vi "Wait.vi"(11 "Time (ms)":u32) -> (3 "Node Out":refnum<class "bt_Node.lvclass">)   [LabVIEW 2021, in "BT.lvlib"]
uses:
  BT.lvlib
  Support/Nodes/abs_Node/bt_Node.lvclass
  Support/Nodes/Leaves/Wait/bt_Wait.lvclass
  C:/Users/Tim/Documents/GitHub/LV_Behaviour_Tree/Source/Support/Nodes/abs_Node/BT_Node.lvclass
  Support/Nodes/Leaves/Wait/bt_Wait.lvclass/bt_Wait.ctl
  Support/Nodes/Leaves/Wait/Properties/Write Time (ms).vi
  C:/Users/Tim/Documents/GitHub/LV_Behaviour_Tree/Source/Support/Nodes/Leaves/Leaf/bt_Leaf.lvclass
  C:/Users/Tim/Documents/GitHub/LV_Behaviour_Tree/Source/Support/Nodes/abs_Node/bt_Node.lvclass
  C:/Users/Tim/Documents/GitHub/LV_Behaviour_Tree/Source/Support/Nodes/Leaves/Wait/bt_Wait.lvclass
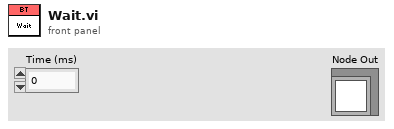
[diagram p1: front panel]
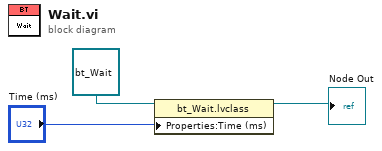
[diagram p0: block diagram]
diagram:
  n1 = property class="bt_Wait.lvclass"(reference=refnum<class "bt_Wait.lvclass"> refnum ("BT.lvlib:Wait.lvclass"), "Properties:Time (ms)"="Time (ms)") -> (reference out=→"Node Out":refnum<class "bt_Wait.lvclass">)  [unwired: 1 in, 1 out]
